vi "NF WF1973_74 Close.vi"(1 "Error In":errorcluster, 2 "VISAsession":refnum<visa-resource-name>) -> (0 "Error Out":errorcluster)   [LabVIEW 2010]
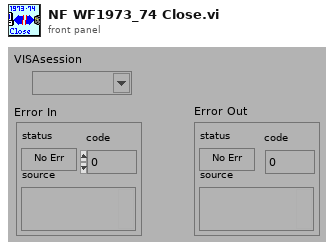
[diagram p1: front panel]
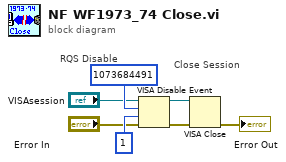
[diagram p0: block diagram]
diagram:
  # "Close Session"
  # "RQS Disable"
  n1 = VISA Disable Event(8:"Error In", 9:u16 1, 10:u32 1073684491, 11:"VISAsession") -> (0:w4:errorcluster, 3:w3:refnum<visa-resource-name>)
  n2 = VISA Close(VISA resource name=w3, error in (no error)=w4) -> (error out=→"Error Out":errorcluster)
